vi "Style String To Bools.vi"(11 "Style String":string) -> (0 "Underlined":bool, 1 "Strikeout":bool, 2 "Italic":bool, 3 "Bold":bool)   [LabVIEW 2021, in "Appearance Actor.lvlib" / "Generic Theme.lvclass"]
doc: "Match style characters (case unsensitive) in <B>Style String</B> and set the corresponding style flag:\n'b': Bold\n'i': Italic\n's' : Strikeout\n'u': Underline"
uses:
  Generic Theme.lvclass
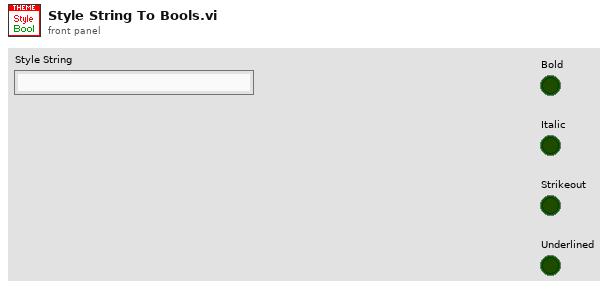
[diagram p1: front panel]
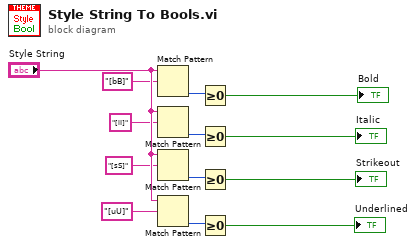
[diagram p0: block diagram]
diagram:
  n1 = Match Pattern(string="Style String", regular expression="[bB]") -> (offset past match=w13:i32)  [unwired: 1 in, 3 out]
  n2 = Match Pattern(string="Style String", regular expression="[iI]") -> (offset past match=w11:i32)  [unwired: 1 in, 3 out]
  n3 = Match Pattern(string="Style String", regular expression="[sS]") -> (offset past match=w9:i32)  [unwired: 1 in, 3 out]
  n4 = Match Pattern(string="Style String", regular expression="[uU]") -> (offset past match=w7:i32)  [unwired: 1 in, 3 out]
  n5 = Greater Or Equal To 0?(x=w13) -> (x >= 0?=→"Bold":bool)
  n6 = Greater Or Equal To 0?(x=w11) -> (x >= 0?=→"Italic":bool)
  n7 = Greater Or Equal To 0?(x=w9) -> (x >= 0?=→"Strikeout":bool)
  n8 = Greater Or Equal To 0?(x=w7) -> (x >= 0?=→"Underlined":bool)
